vi "CAPFM-Analyze.vi"(5 "Control":dbl[](array[numeric]), 7 "Masked":dbl[](array[numeric]), 9 "Index":i32, 11 "error in (no error)":errorcluster, 12 "Analysis":T1) -> (4 "Mags":cluster{"Interval":dbl[], "Control":dbl[]}[](array[cluster]), 8 "Decrement":cluster{"Interval":dbl[], "Decrement":dbl[]}, 14 "Analysis Out":T1, 15 "error out":errorcluster)   [LabVIEW 2020]
uses:
  Typedefs/CAPFM-Analysis State.ctl
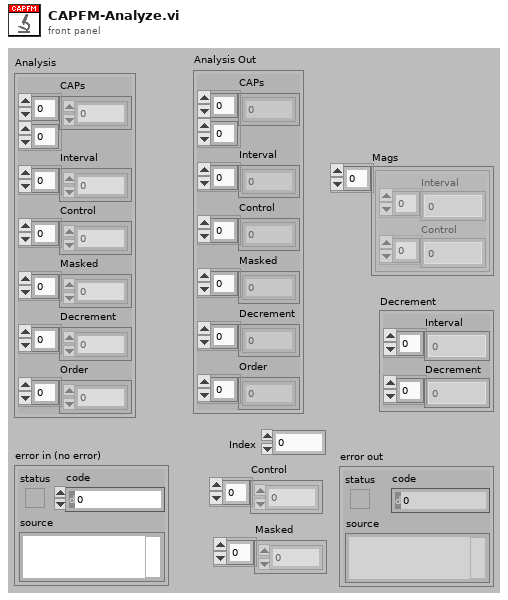
[diagram p1: front panel]
types:
  T1 = typedef "CAPFM-Analysis State.ctl" = cluster{"CAPs":dbl[][], "Interval":dbl[], "Control":dbl[], "Masked":dbl[], "Decrement":dbl[], "Order":i32[]}
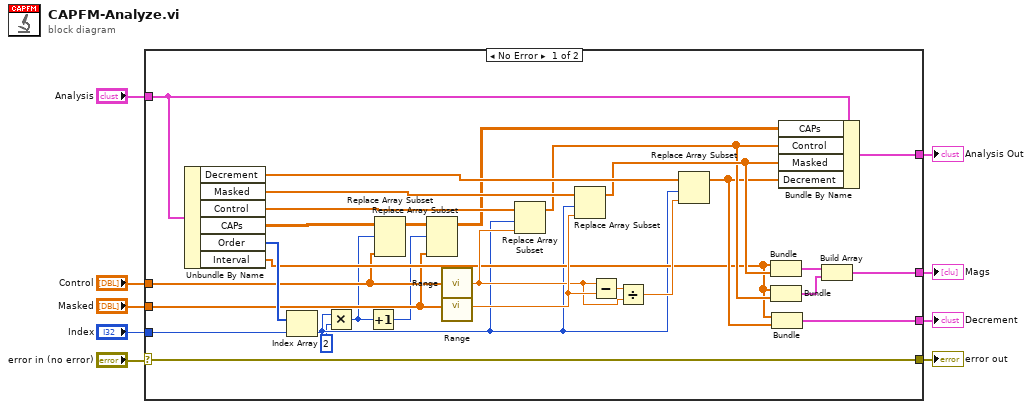
[diagram p0: block diagram]
diagram:
  n1 = case shown="No Error" "error in (no error)" {
    selector: "error in (no error)" -> [w38 w40]
    tunnel: [w38 w40] -> w8
    tunnel: "Analysis" -> [w28 w39]
    tunnel: "Control" -> [w14 _]
    tunnel: "Masked" -> [w17 _]
    tunnel: "Index" -> [w29 _]
    tunnel: [w23 w39] -> w3
    tunnel: [w21 _] -> w2
    tunnel: [w20 _] -> w1
    frame No Error {
      n2 = Unbundle By Name(w28) -> ("Decrement"=w32:dbl[], "Masked"=w36:dbl[], "Control"=w37:dbl[], "CAPs"=w16:dbl[][], "Order"=w30:i32[], "Interval"=w18:dbl[])
      n3 = Index Array(array=w30, index=w29) -> (element=w13:i32)
      n4 = Multiply(x=w13, y=2) -> (x*y=w11:i32)
      n5 = Increment(x=w11) -> (x+1=w10:i32)
      n6 = Replace Array Subset(array=w16, new element=w14, index (row)=w11) -> (w15:dbl[][])  [unwired: 1 in]
      n7 = Replace Array Subset(array=w15, new element=w17, index (row)=w10) -> (w19:dbl[][])  [unwired: 1 in]
      n8 = call "Range.vi"("Array"=w14) -> ("Range"=w33:dbl)
      n9 = call "Range.vi"("Array"=w17) -> ("Range"=w35:dbl)
      n10 = Replace Array Subset(array=w37, new element=w33, index=w13) -> (w26:dbl[])
      n11 = Replace Array Subset(array=w36, new element=w35, index=w13) -> (w27:dbl[])
      n12 = Subtract(x=w33, y=w35) -> (x-y=w34:dbl)
      n13 = Divide(x=w34, y=w33) -> (x/y=w31:dbl)
      n14 = Replace Array Subset(array=w32, new element=w31, index=w13) -> (w25:dbl[])
      n15 = Bundle("Interval"=w18, "Masked"=w27) -> (w24:cluster{"Interval":dbl[], "Masked":dbl[]})  [unwired: 1 in]
      n16 = Bundle("Interval"=w18, "Control"=w26) -> (w22:cluster{"Interval":dbl[], "Control":dbl[]})  [unwired: 1 in]
      n17 = Bundle("Interval"=w18, "Decrement"=w25) -> (w20:cluster{"Interval":dbl[], "Decrement":dbl[]})  [unwired: 1 in]
      n18 = Bundle By Name(cluster=w28, "CAPs"=w19, "Control"=w26, "Masked"=w27, "Decrement"=w25) -> (w23:T1)
      n19 = Build Array(w24, w22) -> (w21:cluster{"Interval":dbl[], "Control":dbl[]}[])
    }
    frame Error {
    }
  }
  "error out" <- w8
  "Analysis Out" <- w3
  "Mags" <- w2
  "Decrement" <- w1
